vi "Find Components Mapping From Component or Channel Name.vi"(10 "module/channel name":string, 11 "module mapping":T1[](array[typedef])) -> (1 "index":i32, 2 "found?":bool, 3 "found mapping":T1)   [LabVIEW 2013, in "Engine Runtime Interface.lvclass"]
uses:
  Engine Runtime Interface.lvclass
  Engine Configuration/Module Mappings.ctl
  <vilib>/NI/Tag Bus/table/mapping specification.ctl
  <vilib>/NI/Tag Bus/tag/Data Type.ctl
  <vilib>/NI/Tag Bus/table/mapping.ctl
  <vilib>/NI/Tag Bus/tag/tag descriptor.lvclass
  Engine Configuration/engine configuration.lvclass
  <vilib>/NI/Tag Bus/table/data table.lvlib
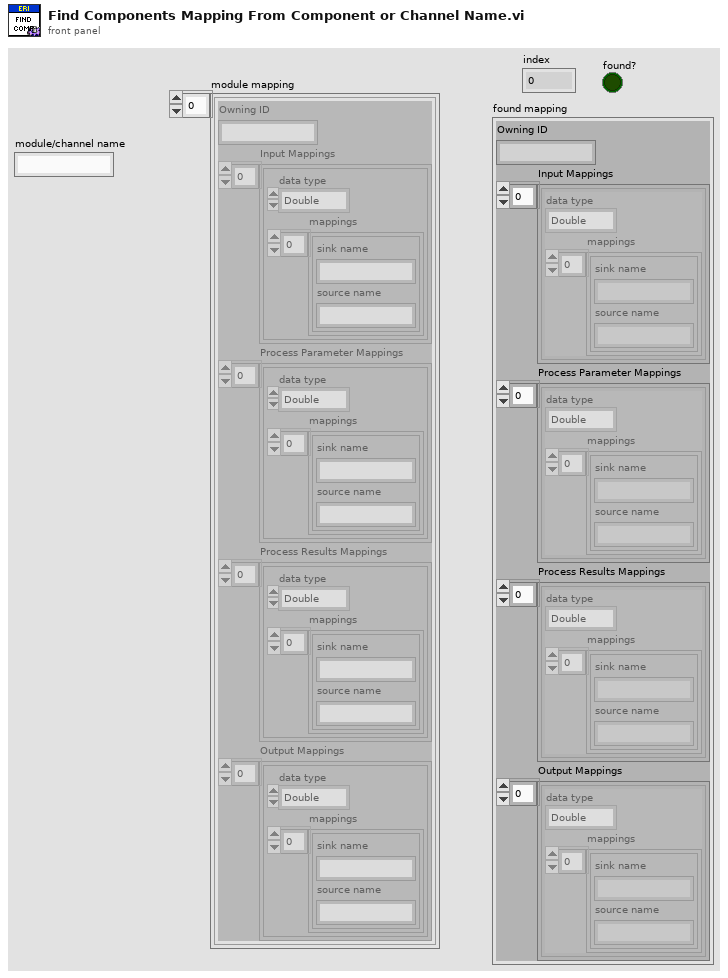
[diagram p1: front panel]
types:
  T1 = typedef "engine configuration.lvclass/Module Mappings.ctl" = cluster{"Owning ID":string, "Input Mappings":T2[], "Process Parameter Mappings":T2[], "Process Results Mappings":T2[], "Output Mappings":T2[]}
  T2 = typedef "tag bus.lvlib/data table.lvlib/mapping specification.ctl" = cluster{"data type":T3, "mappings":T4[]}
  T3 = typedef "tag bus.lvlib/tag descriptor.lvclass/Data Type.ctl" = enum16{"Double", "Single", "I64", "I32", "I16", "I8", "U64", "U32", "U16", "U8", "Boolean", "String", "Array of Double", "Array of Single", "Array of I64", "Array of I32", "Array of I16", "Array of I8", "Array of U64", "Array of U32", "Array of U16", "Array of U8", "Array of Boolean", "Array of String"}
  T4 = typedef "tag bus.lvlib/data table.lvlib/mapping.ctl" = cluster{"sink name":string, "source name":string}
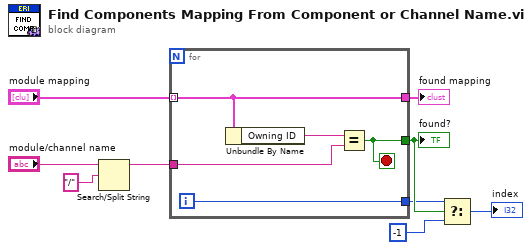
[diagram p0: block diagram]
diagram:
  n1 = Search/Split String(string="module/channel name", search string/char (-)="/") -> (substring before match=w6:string)  [unwired: 1 in, 2 out]
  n2 = for {
    tunnel: "module mapping" -> [w12] mode=indexing
    tunnel: w6 -> [w13]
    tunnel: [w12] -> w5
    tunnel: [w11] -> w3
    tunnel: [w10] -> w2
    i -> [w10]
    stop <- w11 stop-if-true
    n3 = Unbundle By Name(w12) -> ("Owning ID"=w14:string)
    n4 = Equal?(x=w14, y=w13) -> (x = y?=w11:bool)
  }
  "found mapping" <- w5
  "found?" <- w3
  n5 = Select(t=w2, s=w3, f=-1) -> (s? t:f=→"index":i32)
